vi "lvEtherbone.handler_setMap.vi"(0 "eb_socketID":i32, 1 "eb_handlerID":i32, 2 "address":u64 format="%.0x", 4 "data":u8[](array[numeric]), 5 "error in (no error)":errorcluster) -> (13 "eb_status":T1, 14 "eb_socketID out":i32, 15 "eb_handlerID out":i32, 19 "error out":errorcluster)   [LabVIEW 2009, in "lvEtherbone.lvlib"]
doc: "//-----------------------------------------------------------------------------------\n// author : Dietrich Beck, GSI-Darmstadt\n// purpose : Copy data from the \"data\" buffer to the memory map of THIS\n// virtual device. \n// returns : lveb_status_t\n//-----------------------------------------------------------------------------------\nETHERBONE_API int lveb_handler_setMap( int eb_handlerID, //ID of the handler of THIS device\n eb_address_t address, //address where to data is written to\n int size, //size of data to write\n char *data //buffer containing write-data\n );"
uses:
  lvEtherbone.lvlib
  lvEtherbone.lveb_status_t.ctl
  bin/lvEtherbone.dll
panel:
  in  "myeb_status_t":T1
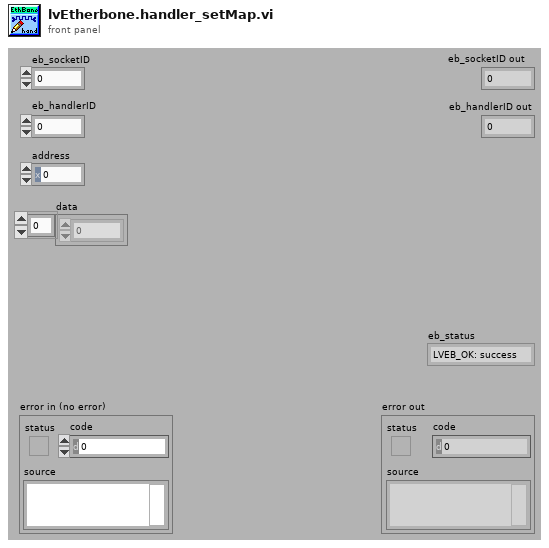
[diagram p1: front panel]
types:
  T1 = typedef "lvEtherbone.lvlib/lvEtherbone.lveb_status_t.ctl" = enum32{"LVEB_OK: success", "LVEB_UNKNOWN: unknown error", "LVEB_OS: operating system forbids access", "LVEB_PORT: port in use or unavailable", "LVEB_ID: ID invalid or out of resources", "LVEB_SOCKET: socket invalid or unavailable", "LVEB_EB: remote address is not Etherbone conformant", "LVEB_IP: bad format or network address", "LVEB_BUSWIDTH: bus width error", "LVEB_DEVICEBUSY: Whishbone device still busy", "LVEB_DEVICEFAIL: operation on Wishbone device failed", "LVEB_DEVICEEXIST: Whishbone device already exists, overlaps, or does not exist", "LVEB_TIMEDOUT: a timeout occurred", "LVEB_OVERFLOW: payload of Etherbone exceeded", "LVEB_ADDRESS: bad address"}
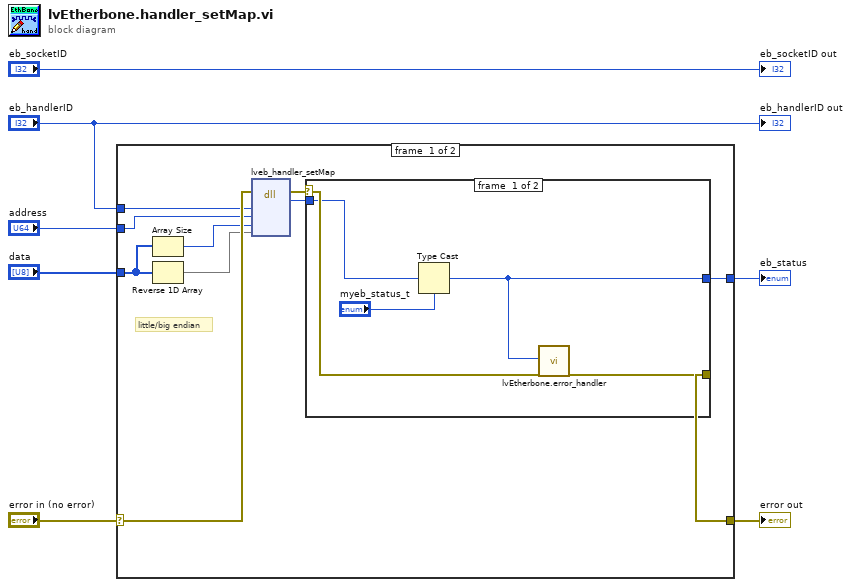
[diagram p0: block diagram]
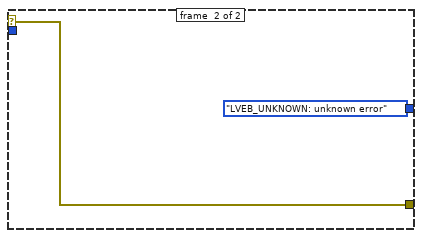
[diagram p2: hidden frame]
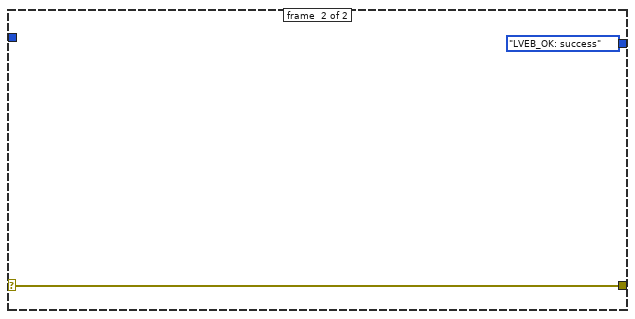
[diagram p3: hidden frame]
diagram:
  n1 = case shown="No Error" "error in (no error)" {
    selector: "error in (no error)" -> [w17 w26]
    tunnel: [w13 w26] -> w6
    tunnel: "eb_handlerID" -> [w16 _]
    tunnel: [w12 lvEtherbone.lveb_status_t."LVEB_OK: success" ("eb_status_t")] -> w5
    tunnel: "address" -> [w11 _]
    tunnel: "data" -> [w10 _]
    frame #0 {
      # "little/big endian"
      n2 = Array Size(array=w10) -> (size(s)=w9:i32)
      n3 = Reverse 1D Array(array=w10) -> (reversed array=w8:u8[])
      n4 = dll-call lib="F:/beck/Project/BEL/SCC/etherbone-core/api/lvEtherbone/bin/lvEtherbone.*" fn="lveb_handler_setMap"(error in=w17, "eb_handlersID"=w16, "address"=w11, "size"=w9, "data"=w8) -> (error out=w15:errorcluster, "myeb_status"=w14:i32)  [unwired: 6 in, 1 out]
      n5 = case shown="No Error" w15 {
        selector: w15 -> [w21 w24]
        tunnel: w14 -> [w20 _]
        tunnel: [w19 lvEtherbone.lveb_status_t."LVEB_UNKNOWN: unknown error" ("eb_status_t")] -> w12
        tunnel: [w22 w24] -> w13
        frame #0 {
          n6 = Type Cast(type="myeb_status_t", x=w20) -> (*(type *) &x=w19:T1)
          n7 = call "lvEtherbone.error_handler.vi"("eb_status"=w19, "error in"=w21) -> ("error out"=w22:errorcluster)  [unwired: 17 in]
        }
        frame #1 {
        }
      }
    }
    frame #1 {
    }
  }
  "error out" <- w6
  "eb_status" <- w5
  "eb_socketID out" <- "eb_socketID"
  "eb_handlerID out" <- "eb_handlerID"
